vi "Monitor-ConvertRectToSquare.vi"(10 "Rect coords in":T1) -> (2 "Square coords out":T1)   [LabVIEW 2016]
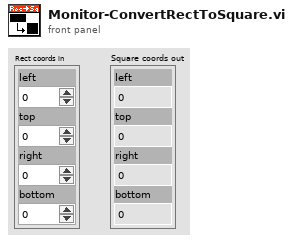
[diagram p1: front panel]
types:
  T1 = cluster{"left":i16, "top":i16, "right":i16, "bottom":i16}
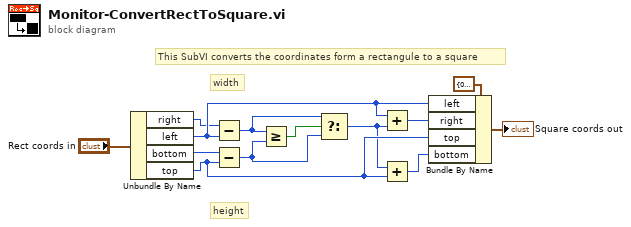
[diagram p0: block diagram]
diagram:
  # "width"
  # "height"
  # "This SubVI converts the coordinates form a rectangule to a square"
  n1 = Unbundle By Name("Rect coords in") -> ("right"=w10:i16, "left"=w12:i16, "bottom"=w11:i16, "top"=w13:i16)
  n2 = Subtract ("Width")(x=w10, y=w12) -> (x-y=w6:i16)
  n3 = Subtract ("Height")(x=w11, y=w13) -> (x-y=w5:i16)
  n4 = Greater Or Equal?(x=w6, y=w5) -> (x >= y?=w7:bool)
  n5 = Select(t=w6, s=w7, f=w5) -> (s? t:f=w2:i16)
  n6 = Add(x=w12, y=w2) -> (x+y=w1:i16)
  n7 = Add(x=w2, y=w13) -> (x+y=w3:i16)
  n8 = Bundle By Name(cluster=T1 {"left"=0, "top"=0, "right"=0, "bottom"=0} ("rect"), "left"=w12, "right"=w1, "top"=w13, "bottom"=w3) -> (→"Square coords out":T1)
